vi "Get File Extension.vi"(0 "file path in":path=path "C:/Users/vs/Desktop/Get File Extension.vi" caption="文件", 1 "error IO":errorcluster) -> (2 "file path out":path=path "C:/Users/vs/Desktop/Get File Extension.vi" caption="文件副本", 3 "unmodified file extension":string="vi" caption="未改动的文件扩展名", 4 "filename without extension":string="Get File Extension" caption="无扩展名的文件名", 5 "error IO 2":errorcluster caption="error IO")   [LabVIEW 2014]
doc: "返回指定文件的文件扩展名，不包括句点(.)。"
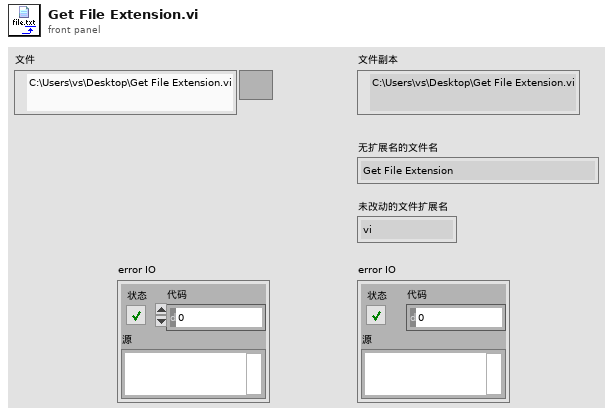
[diagram p1: front panel]
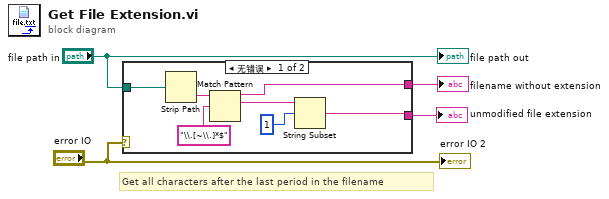
[diagram p0: block diagram]
diagram:
  # "Get all characters after the last period in the filename"
  n1 = case shown="无错误" "error IO" {
    tunnel: "file path in" -> [w10 _]
    tunnel: [w6 _] -> w3
    tunnel: [w5 _] -> w2
    frame No Error {
      n2 = Strip Path(path=w10) -> (name=w9:string)  [unwired: 1 out]
      n3 = Match Pattern(string=w9, regular expression="\\.[~\\.]*$") -> (before substring=w6:string, match substring=w11:string)  [unwired: 3 out]
      n4 = String Subset(string=w11, offset (0)=1) -> (substring=w5:string)  [unwired: 1 out]
    }
    frame Error {
    }
  }
  "filename without extension" <- w3
  "unmodified file extension" <- w2
  "file path out" <- "file path in"
  "error IO 2" <- "error IO"
